vi "gc-zyklus mfc konfig.vi"() -> ()   [LabVIEW 2010]
uses:
  <vilib>/Instr/_visa.llb/VISA Configure Serial Port (Instr).vi
panel:
  in  "Konfigurationsdatei auswählen":path
  out "Konfiguration":string
  out "Zeitpunkt":string
  out "Temperatur (°C)":u16
  out "Meßwert PC2 (mbara)":u16
  out "Meßwert PC1 (mbara)":u16
  out "Meßwert FC (mln/min)":u16
  in  "Setpoint PC1 (bara)":dbl min=0.15 max=3.0 step=0.05
  in  "Setpoint PC2 (bara)":dbl min=0.15 max=3.0 step=0.05
  in  "Messwerte speichern":path
  out "Zyklus Nr.":i32
  out "Positionen (1-6)":i32[](array[numeric])=[1, 3, 5, 2]
  out "Anzahl der Zustände (Mpos.-Ventil)":i32
  out "aktuelle Position":i32
  out "Setpoints FC (ln/min)":dbl[](array[numeric])=[1.0, 3.0, 5.0, 2.0]
  out "Längen der Zustände (s)":i32[](array[numeric])=[1, 3, 5, 2]
  out "Anzahl der Zustände (MFC)":i32
  out "Länge des aktuellen Zustandes (s)":i32
  out "aktueller Setpoint FC (ln/min)":dbl
  out "Sequenz Nr.":i32
  out "Aktuelle Zeit":timestamp
  in  "(Sequenz wird zu Ende geführt)":bool
  # "Gerät im Chromatographie-Zyklus, z.B. MFC"
  # "Multipositionsventil"
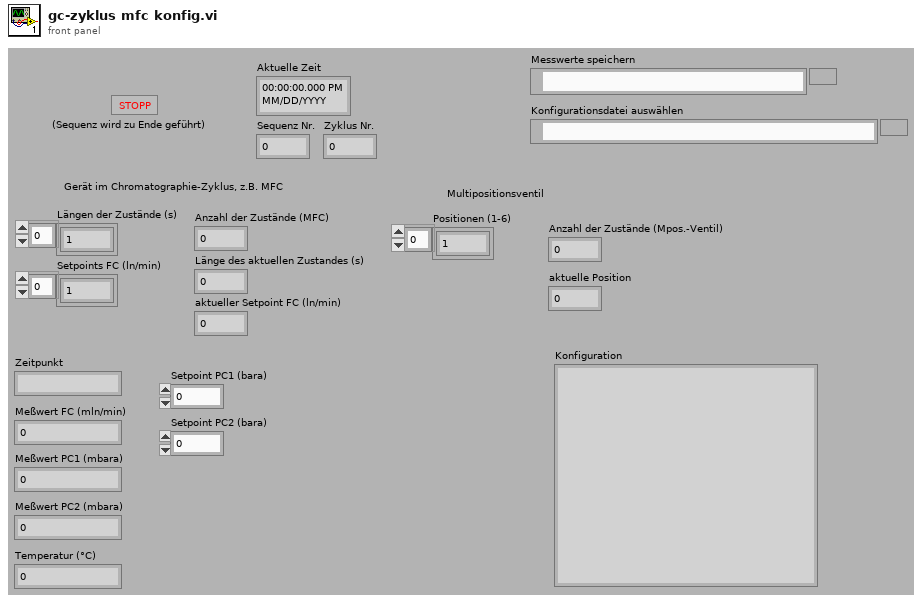
[diagram p1: front panel]
types:
  T1 = enum16{"open", "replace", "create", "open or create", "replace or create", "replace or create with confirmation"}
  T2 = cluster{"Mode":enum16{"RTU", "ASCII"}, "Slave Address":u8}
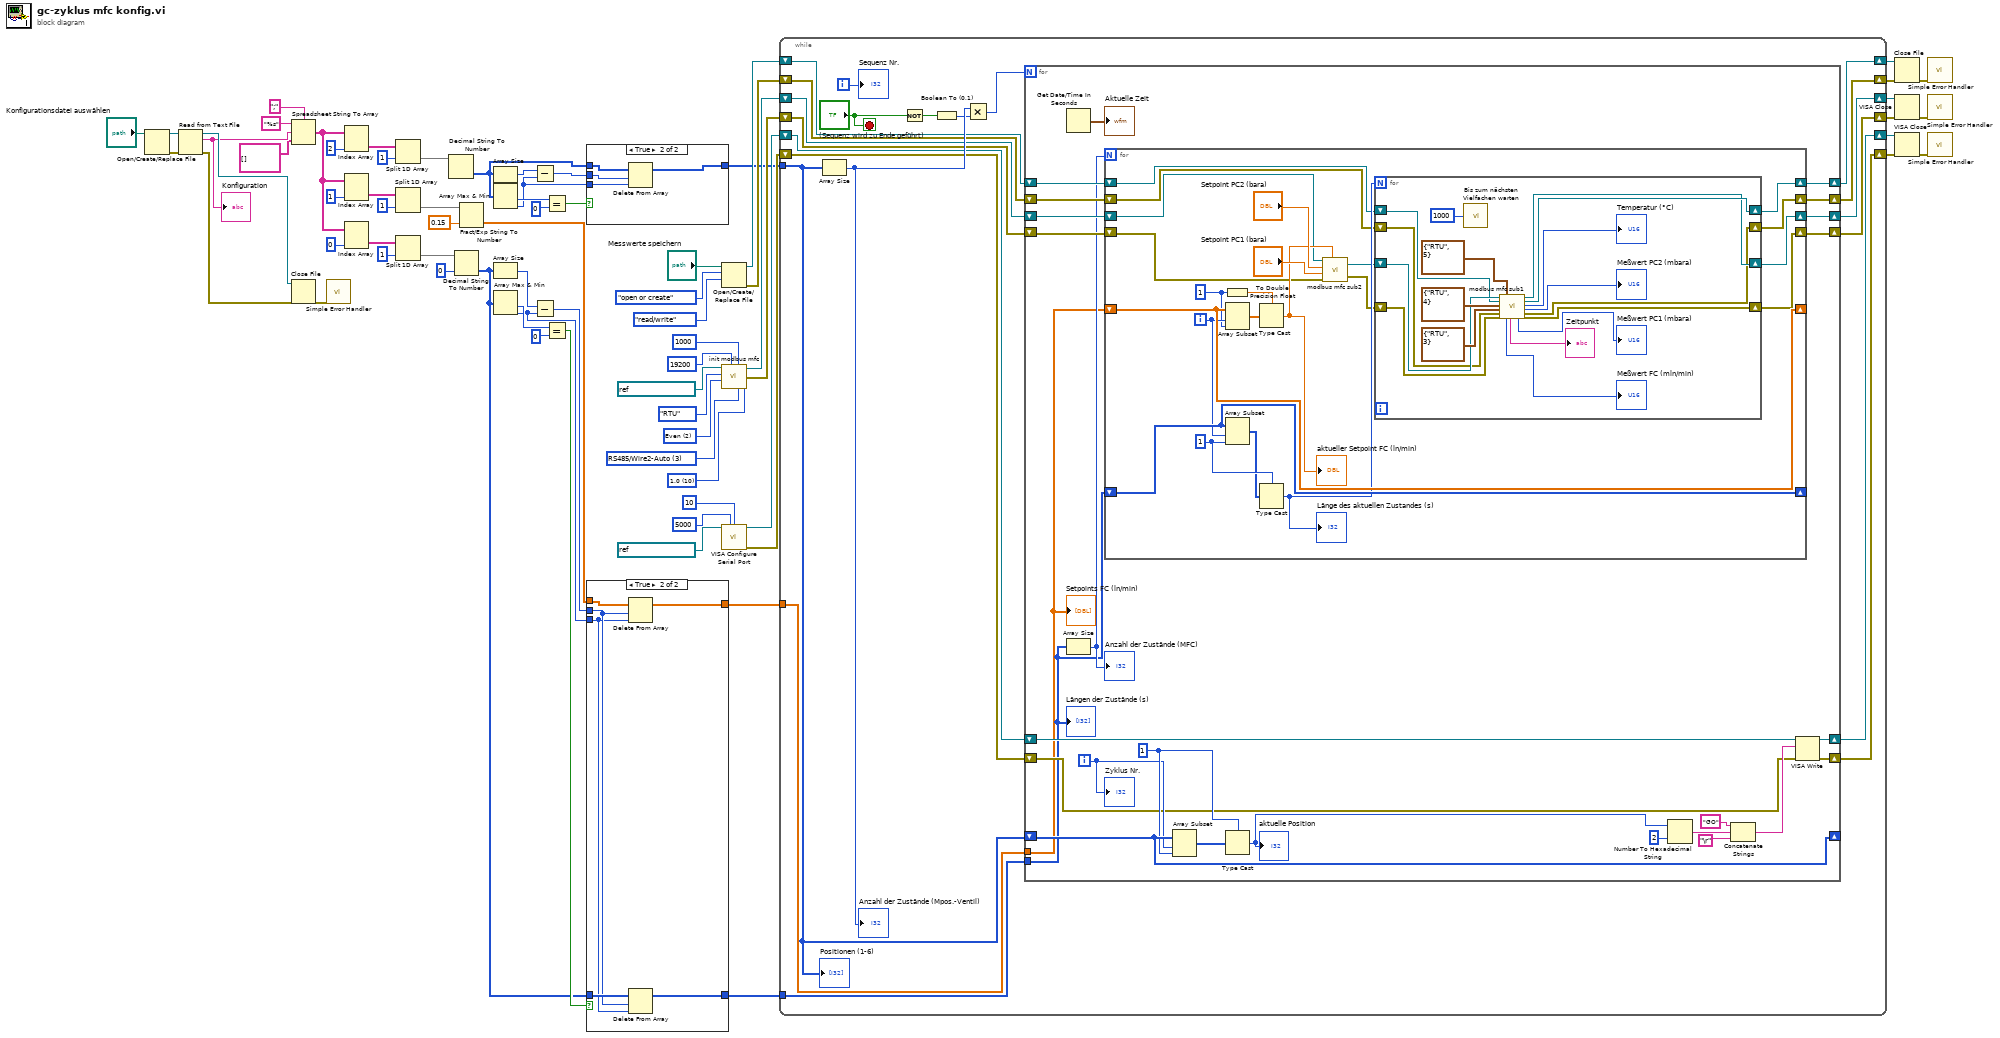
[diagram p0: block diagram]
diagram:
  w68 = u16 10 items=["1.0"=10, "1.5"=15, "2.0"=20] ("Serial Settings:Stop Bits")
  w66 = u16 2 items=["None", "Odd", "Even", "Mark", "Space"] ("Parity")
  w67 = i16 3 items=["Unknown"=-1, "RS485/Wire4"=0, "RS485/Wire2-EchoDTR"=1, "RS485/Wire2-CtrlDTR"=2, "RS485/Wire2-Auto"=3, "RS232/DTE"=128, "RS232/DCE"=129, "RS232/AUTO"=130] ("Serial Settings:Wire Mode")
  n1 = Open/Create/Replace File(file path (use dialog)="Konfigurationsdatei auswählen") -> (refnum out=w43:refnum<file>, error out=w42:errorcluster)  [unwired: 5 in, 1 out]
  n2 = Read from Text File(file (use dialog)=w43, error in=w42) -> (refnum out=w40:refnum<file>, text=w37:string, error out=w41:errorcluster)  [unwired: 2 in, 1 out]
  "Konfiguration" <- w37
  n3 = Spreadsheet String To Array(delimiter (Tab)=";", format string="%s" ("Format-String"), spreadsheet string=w37, array type (2D Dbl)=string[][] []) -> (array=w9:string[][])
  n4 = Close File(refnum=w40, error in=w41) -> (error out=w39:errorcluster)  [unwired: 1 out]
  n5 = call <vilib>:"Simple Error Handler.vi"("error in (no error)"=w39) -> ()  [unwired: 4 in, 5 out]
  n6 = Index Array(array=w9, index (col)=2 ("Index")) -> (element=w21:string[])  [unwired: 1 in]
  n7 = Index Array(array=w9, index (col)=1 ("Index")) -> (element=w15:string[])  [unwired: 1 in]
  n8 = Index Array(array=w9, index (col)=0 ("Index")) -> (element=w11:string[])  [unwired: 1 in]
  n9 = Split 1D Array(array=w21, index=1 ("Index")) -> (second subarray=w19:string[])  [unwired: 1 out]
  n10 = Split 1D Array(array=w15, index=1 ("Index")) -> (second subarray=w13:string[])  [unwired: 1 out]
  n11 = Split 1D Array(array=w11, index=1 ("Index")) -> (second subarray=w6:string[])  [unwired: 1 out]
  n12 = Decimal String To Number(string=w19) -> (number=w23:i32[])  [unwired: 2 in, 1 out]
  n13 = Decimal String To Number(string=w6, default (0L)=0 ("Standard (0 I32)")) -> (number=w25:i32[])  [unwired: 1 in, 1 out]
  n14 = Fract/Exp String To Number(string=w13, default (0 dbl)=0.15 ("Standard (0 DBL)")) -> (number=w24:dbl[])  [unwired: 2 in, 1 out]
  n15 = Array Size(array=w23) -> (size(s)=w18:i32)
  n16 = Array Max & Min(array=w23) -> (min value=w33:i32, min index (indices)=w17:i32)  [unwired: 2 out]
  n17 = Array Size(array=w25) -> (size(s)=w8:i32)
  n18 = Array Max & Min(array=w25) -> (min value=w29:i32, min index (indices)=w7:i32)  [unwired: 2 out]
  n19 = Subtract(x=w18, y=w17) -> (x-y=w30:i32)
  n20 = Subtract(x=w8, y=w7) -> (x-y=w26:i32)
  n21 = Equal?(x=w33, y=0) -> (x = y?=w31:bool)
  n22 = Equal?(x=w29, y=0) -> (x = y?=w27:bool)
  n23 = case shown="True" w31 {
    tunnel: w23 -> [w72 w76]
    tunnel: w17 -> [_ w74]
    tunnel: [w72 w75] -> w5
    tunnel: w30 -> [_ w73]
    frame False {
    }
    frame True {
      n24 = Delete From Array(array=w76, length=w73, index=w74) -> (array with subset deleted=w75:i32[])  [unwired: 1 out]
    }
  }
  n25 = case shown="True" w27 {
    tunnel: w25 -> [w78 w84]
    tunnel: w7 -> [_ w79]
    tunnel: [w78 w83] -> w3
    tunnel: w26 -> [_ w80]
    tunnel: w24 -> [w77 w82]
    tunnel: [w77 w81] -> w4
    frame False {
    }
    frame True {
      n26 = Delete From Array(array=w82, length=w80, index=w79) -> (array with subset deleted=w81:dbl[])  [unwired: 1 out]
      n27 = Delete From Array(array=w84, length=w80, index=w79) -> (array with subset deleted=w83:i32[])  [unwired: 1 out]
    }
  }
  n28 = Open/Create/Replace File(file path (use dialog)="Messwerte speichern", operation (0:open)=T1."open or create" ("Operation (0:Öffnen)"), access (0:read/write)=enum16{"read/write", "read-only", "write-only"}."read/write" ("Zugriff (0:Lesen/Schreiben)")) -> (refnum out=w61:refnum<file>, error out=w60:errorcluster)  [unwired: 3 in, 1 out]
  n29 = call "init modbus mfc.vi"("Timeout"=u32 1000, "Serial Settings:Stop Bits"=w68, "Serial Settings:Wire Mode"=w67, "Baud Rate"=u32 19200, "VISA resource name"=refnum<visa-resource-name> "ASRL2::INSTR", "Mode"=enum16{"RTU", "ASCII"}."RTU", "Parity"=w66) -> ("VISA resource name out"=w59:refnum<visa-resource-name>, "error out"=w58:errorcluster)  [unwired: 2 in]
  n30 = call-poly "VISA Configure Serial Port"("VISA resource name"=refnum<visa-resource-name> "ASRL1::INSTR", "timeout (10sec)"=u32 5000, "termination char\n(0xA = '\\n' = LF)"=u8 10 ("termination char\n(0xA = '\\n' = LF)")) -> ("VISA resource name out"=w48:refnum<visa-resource-name>, "error out"=w47:errorcluster)  [unwired: 11 in]
  n31 = while {
    shift-right: [w95] -> w52
    shift-left: w61 -> [w99]
    shift-right: [w94] -> w51
    shift-left: w60 -> [w98]
    shift-right: [w93] -> w50
    shift-left: w59 -> [w97]
    shift-right: [w92] -> w49
    shift-left: w58 -> [w96]
    shift-right: [w89] -> w45
    shift-left: w48 -> [w91]
    shift-right: [w88] -> w44
    shift-left: w47 -> [w90]
    tunnel: w5 -> [w87]
    tunnel: w4 -> [w86]
    tunnel: w3 -> [w85]
    i -> [w105]
    stop <- "(Sequenz wird zu Ende geführt)" stop-if-true
    n32 = Array Size(array=w87) -> (size(s)=w104:i32)
    "Anzahl der Zustände (Mpos.-Ventil)" <- w104
    n33 = Not(x="(Sequenz wird zu Ende geführt)") -> (.not. x?=w102:bool)
    n34 = Boolean To (0,1)(Boolean=w102) -> (0, 1=w100:i16)
    n35 = Multiply(x=w104, y=w100) -> (x*y=w101:i32)
    n36 = for {
      N: w101 -> [_]
      shift-right: [w131] -> _
      shift-left: w87 -> [w131]
      shift-right: [w115] -> w95
      shift-left: w99 -> [w123]
      shift-right: [w114] -> w94
      shift-left: w98 -> [w124]
      shift-right: [w113] -> w93
      shift-left: w97 -> [w126]
      shift-right: [w112] -> w92
      shift-left: w96 -> [w125]
      shift-right: [w109] -> w89
      shift-left: w91 -> [w111]
      shift-right: [w108] -> w88
      shift-left: w90 -> [w110]
      tunnel: w86 -> [w107]
      tunnel: w85 -> [w106]
      i -> [w128]
      w130 = 1 ("Länge")
      n37 = Get Date/Time In Seconds() -> (seconds since 1Jan1904=→"Aktuelle Zeit":timestamp)
      n38 = Array Size(array=w106) -> (size(s)=w122:i32)
      "Anzahl der Zustände (MFC)" <- w122
      n39 = for {
        N: w122 -> [_]
        shift-right: [w153] -> _
        shift-left: w106 -> [w153]
        shift-right: [w149] -> _
        shift-left: w107 -> [w149]
        shift-right: [w142] -> w115
        shift-left: w123 -> [w143]
        shift-right: [w140] -> w114
        shift-left: w124 -> [w144]
        shift-right: [w141] -> w113
        shift-left: w126 -> [w135]
        shift-right: [w139] -> w112
        shift-left: w125 -> [w134]
        i -> [w148]
        w146 = 1 ("Länge")
        w152 = 1 ("Länge")
        n40 = To Double Precision Float(number=w146) -> (double precision float=w145:dbl)
        n41 = Array Subset(array=w149, index=w148, length=w146) -> (w150:dbl[])
        n42 = Array Subset(array=w153, index=w148, length=w152) -> (w151:i32[])
        n43 = Type Cast(type=w145, x=w150) -> (*(type *) &x=w136:dbl)
        "aktueller Setpoint FC (ln/min)" <- w136
        n44 = Type Cast(type=w152, x=w151) -> (*(type *) &x=w147:i32)
        "Länge des aktuellen Zustandes (s)" <- w147
        n45 = call "modbus mfc sub2.vi"("VISA resource name out 2"=w135, "Setpoint PC2 (bara)"="Setpoint PC2 (bara)", "Setpoint PC1 (bara)"="Setpoint PC1 (bara)", "error out 2"=w134, "Setpoint FC (ln/min)"=w136) -> ("VISA resource name out"=w133:refnum<visa-resource-name>, "error out"=w132:errorcluster)
        n46 = for {
          N: w147 -> [_]
          shift-right: [w156] -> w141
          shift-left: w133 -> [w160]
          shift-right: [w157] -> w142
          shift-left: w143 -> [w158]
          shift-right: [w155] -> w140
          shift-left: w144 -> [w159]
          shift-right: [w154] -> w139
          shift-left: w132 -> [w161]
          n47 = call "Bis zum nächsten Vielfachen warten"("Count(mSec)"=u32 1000) -> ()  [unwired: 1 out]
          n48 = call "modbus mfc sub1.vi"("VISA resource name out"=w160, "refnum out 2"=w158, "Serial Parameters 2"=T2 {"Mode"=enum."RTU", "Slave Address"=4}, "Serial Parameters"=T2 {"Mode"=enum."RTU", "Slave Address"=3}, "error out 2"=w159, "error out 3"=w161, "Serial Parameters 3"=T2 {"Mode"=enum."RTU", "Slave Address"=5}) -> ("Numerisch 3"=→"Meßwert FC (mln/min)":u16, "date/time string"=→"Zeitpunkt":string, "Numerisch 2"=→"Meßwert PC1 (mbara)":u16, "VISA resource name out 2"=w156:refnum<visa-resource-name>, "refnum out"=w157:refnum<file>, "Numerisch 4"=→"Temperatur (°C)":u16, "Numerisch"=→"Meßwert PC2 (mbara)":u16, "error out"=w155:errorcluster, "error out 4"=w154:errorcluster)  [unwired: 3 in, 1 out]
        }
      }
      n49 = Array Subset(array=w131, index=w128, length=w130) -> (w129:i32[])
      n50 = Type Cast(type=w130, x=w129) -> (*(type *) &x=w116:i32)
      "aktuelle Position" <- w116
      n51 = Number To Hexadecimal String(1:i16 2 ("Breite (-)"), 2:w116) -> (0:w120:string)
      n52 = Concatenate Strings("GO" ("String"), w120, "\r") -> (w121:string)
      n53 = VISA Write(VISA resource name=w111, write buffer=w121, error in (no error)=w110) -> (VISA resource name out=w109:refnum<visa-resource-name>, error out=w108:errorcluster)  [unwired: 1 out]
      "Längen der Zustände (s)" <- w106
      "Setpoints FC (ln/min)" <- w107
      "Zyklus Nr." <- w128
    }
    "Positionen (1-6)" <- w87
    "Sequenz Nr." <- w105
  }
  n54 = Close File(refnum=w52, error in=w51) -> (error out=w56:errorcluster)  [unwired: 1 out]
  n55 = VISA Close(VISA resource name=w50, error in (no error)=w49) -> (error out=w57:errorcluster)
  n56 = VISA Close(VISA resource name=w45, error in (no error)=w44) -> (error out=w46:errorcluster)
  n57 = call <vilib>:"Simple Error Handler.vi"("error in (no error)"=w56) -> ()  [unwired: 4 in, 5 out]
  n58 = call <vilib>:"Simple Error Handler.vi"("error in (no error)"=w57) -> ()  [unwired: 4 in, 5 out]
  n59 = call <vilib>:"Simple Error Handler.vi"("error in (no error)"=w46) -> ()  [unwired: 4 in, 5 out]
